vi "Get Name.vi"(8 "error in (no error)":errorcluster, 11 "Generic Plugin in":refnum<class "Generic Plugin.lvclass">) -> (0 "error out":errorcluster, 2 "Get Name":string, 3 "Generic Plugin out":refnum<class "Generic Plugin.lvclass">)   [LabVIEW 2019, in "Generic Plugin.lvclass"]
uses:
  Generic Plugin.lvclass
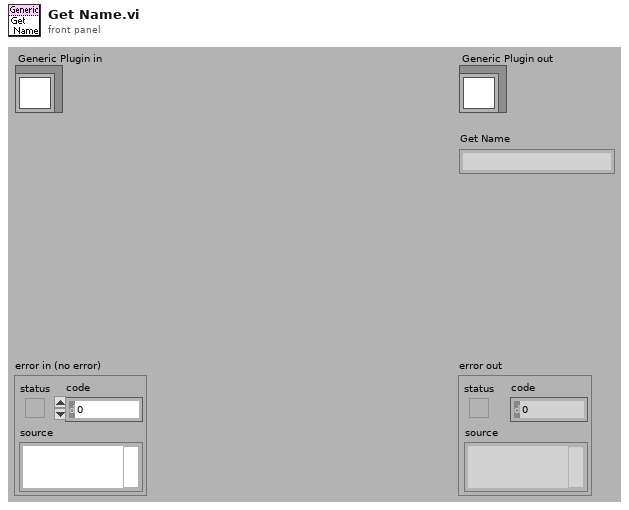
[diagram p1: front panel]
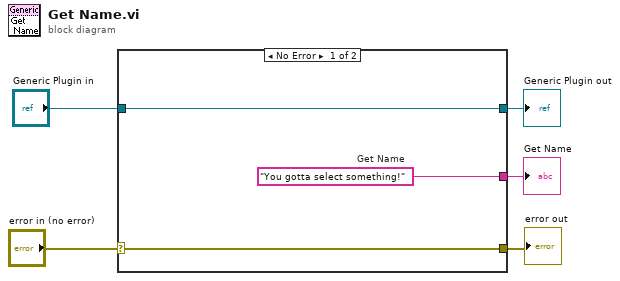
[diagram p0: block diagram]
diagram:
  n1 = case shown="No Error" "error in (no error)" {
    selector: "error in (no error)" -> [w7 w10]
    tunnel: [w7 w10] -> w4
    tunnel: [w8 w9] -> w2
    tunnel: "Generic Plugin in" -> [w8 w9]
    tunnel: [w6 _] -> w1
    frame No Error {
      w6 = "You gotta select something!"  # Get Name
    }
    frame Error {
    }
  }
  "error out" <- w4
  "Generic Plugin out" <- w2
  "Get Name" <- w1
